vi "updateEndTime.vi"(8 "error in (no error)":errorcluster, 11 "RampEvent in":refnum<class "RampEvent.lvclass">) -> (0 "error out":errorcluster, 3 "RampEvent out":refnum<class "RampEvent.lvclass">)   [LabVIEW 2009, in "Tools.lvlib" / "Scripting.lvlib" / "RampEvent.lvclass"]
uses:
  RampEvent.lvclass
  RampEvent.lvclass/RampEvent.ctl
  ScriptEvent.lvclass
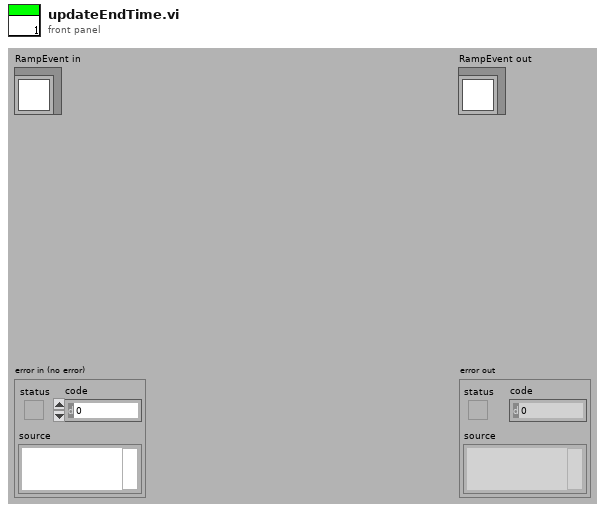
[diagram p1: front panel]
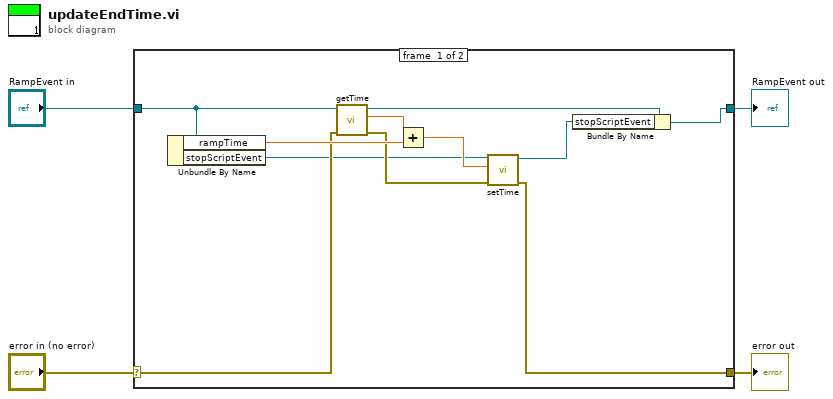
[diagram p0: block diagram]
diagram:
  n1 = case shown="No Error" "error in (no error)" {
    selector: "error in (no error)" -> [w10 w17]
    tunnel: [w6 w17] -> w3
    tunnel: [w5 w16] -> w1
    tunnel: "RampEvent in" -> [w15 w16]
    frame #0 {
      n2 = Unbundle By Name(w15) -> ("rampTime"=w13:dbl, "stopScriptEvent"=w9:refnum<class "ScriptEvent.lvclass">)
      n3 = call "getTime.vi"("error in (no error)"=w10, "ScriptEvent.lvclass in"=w15) -> ("error out"=w11:errorcluster, "time"=w14:dbl, "ScriptEvent.lvclass out"=w8:refnum<class "RampEvent.lvclass">)  [unwired: 7 in]
      n4 = Add(x=w14, y=w13) -> (x+y=w12:dbl)
      n5 = call "setTime.vi"("error in (no error)"=w11, "time"=w12, "ScriptEvent.lvclass in"=w9) -> ("error out"=w6:errorcluster, "ScriptEvent.lvclass out"=w7:refnum<class "ScriptEvent.lvclass">)  [unwired: 7 in]
      n6 = Bundle By Name(cluster=w8, "stopScriptEvent"=w7) -> (w5:refnum<class "RampEvent.lvclass">)
    }
    frame #1 {
    }
  }
  "error out" <- w3
  "RampEvent out" <- w1
